vi "List Rules as Strings.vi"(8 "error in (no error)":errorcluster, 11 "GlobalLogFilter in":refnum<class "GlobalLogFilter.lvclass">) -> (0 "error out":errorcluster, 2 "Rule Strings":string[](array[string]), 3 "GlobalLogFilter out":refnum<class "GlobalLogFilter.lvclass">)   [LabVIEW 2017, in "GlobalLogFilter.lvclass"]
uses:
  GlobalLogFilter.lvclass
  GlobalLogFilter.lvclass/GlobalLogFilter.ctl
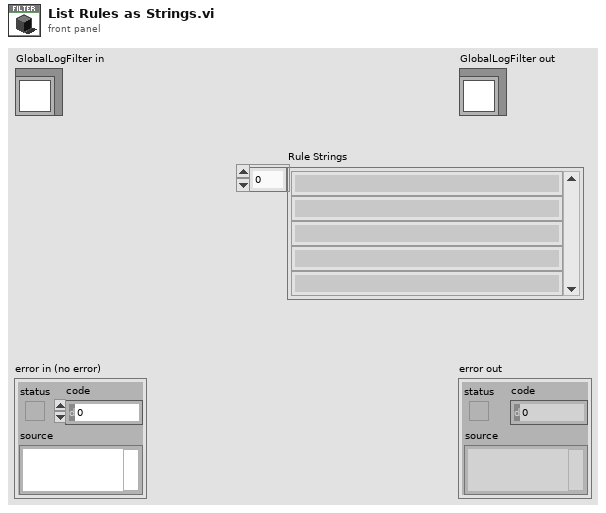
[diagram p1: front panel]
types:
  T1 = typedef "Communicable State Machine.lvlib/_CSM_GlobalLog_MSG_TYPE.ctl" = enum16{"User Log", "State Change", "Status", "Interrupt", "Register", "Unregister", "Error Log", "Module Created", "Module Destroyed"}
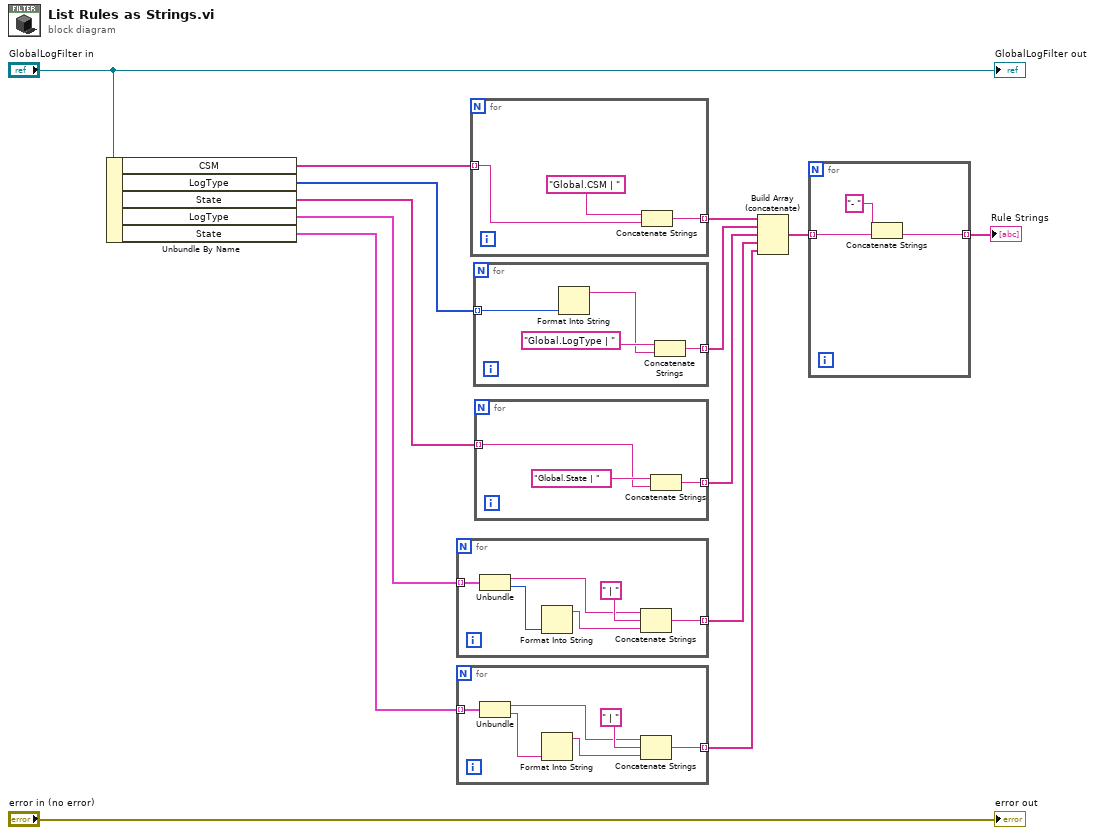
[diagram p0: block diagram]
diagram:
  n1 = Unbundle By Name("GlobalLogFilter in") -> ("CSM"=w12:string[], "LogType"=w10:T1[], "State"=w8:string[], "LogType"=w6:cluster{"CSM":string, "LogType":T1}[], "State"=w4:cluster{"CSM":string, "State":string}[])
  n2 = for {
    tunnel: w6 -> [w18] mode=indexing
    tunnel: [w19] -> w5 mode=indexing
    n3 = Unbundle(w18) -> ("CSM"=w17:string, "LogType"=w16:T1)
    n4 = Format Into String(w16) -> (resulting string=w15:string)  [unwired: 3 in, 1 out]
    n5 = Concatenate Strings(w17, " | " ("string"), w15) -> (w19:string)
  }
  n6 = for {
    tunnel: w4 -> [w24] mode=indexing
    tunnel: [w25] -> w3 mode=indexing
    n7 = Unbundle(w24) -> ("CSM"=w23:string, "State"=w22:string)
    n8 = Format Into String(w22) -> (resulting string=w21:string)  [unwired: 3 in, 1 out]
    n9 = Concatenate Strings(w23, " | " ("string"), w21) -> (w25:string)
  }
  n10 = for {
    tunnel: w12 -> [w28] mode=indexing
    tunnel: [w27] -> w11 mode=indexing
    n11 = Concatenate Strings("Global.CSM | " ("string"), w28) -> (w27:string)
  }
  n12 = for {
    tunnel: w10 -> [w31] mode=indexing
    tunnel: [w32] -> w9 mode=indexing
    n13 = Format Into String(w31) -> (resulting string=w30:string)  [unwired: 3 in, 1 out]
    n14 = Concatenate Strings("Global.LogType | " ("string"), w30) -> (w32:string)
  }
  n15 = for {
    tunnel: w8 -> [w34] mode=indexing
    tunnel: [w35] -> w7 mode=indexing
    n16 = Concatenate Strings("Global.State | " ("string"), w34) -> (w35:string)
  }
  n17 = Build Array (concatenate)(w11, w9, w7, w5, w3) -> (w1:string[])
  n18 = for {
    tunnel: [w37] -> w2 mode=indexing
    tunnel: w1 -> [w38] mode=indexing
    n19 = Concatenate Strings("- " ("string"), w38) -> (w37:string)
  }
  "Rule Strings" <- w2
  "error out" <- "error in (no error)"
  "GlobalLogFilter out" <- "GlobalLogFilter in"
